vi "Get LV Color.vi"(8 "error in (no error)":errorcluster, 11 "Color in":refnum<class "Color.lvclass">) -> (0 "error out":errorcluster, 2 "Color":u32(colorbox), 3 "Color out":refnum<class "Color.lvclass">)   [LabVIEW 2018, in "Color.lvclass"]
doc: "A method to get the LabVIEW color value corresponding the current color."
uses:
  Color.lvclass
panel:
  # "expressionflow.com"
  # "Copyright (c) 2008 Tomi Maila. All rights reserved."
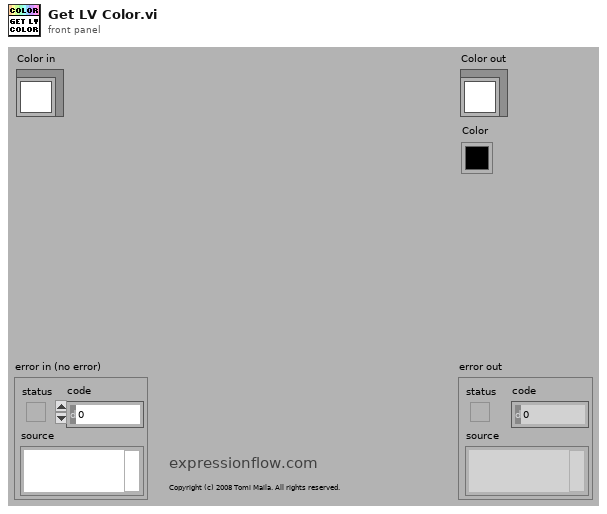
[diagram p1: front panel]
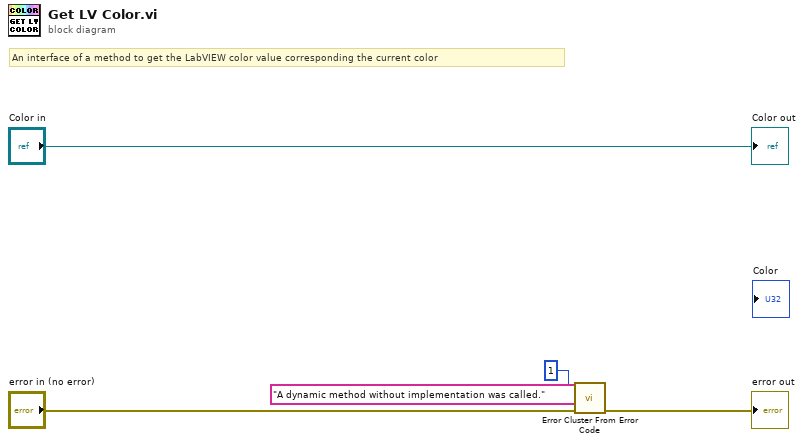
[diagram p0: block diagram]
diagram:
  # "An interface of a method to get the LabVIEW color value corresponding the current color"
  n1 = call <vilib>:"Error Cluster From Error Code.vi"("error in (no error)"="error in (no error)", "error message (\"\")"="A dynamic method without implementation was called." ("error message (\"\")"), "error code (0)"=1) -> ("error out"=→"error out":errorcluster)  [unwired: 6 in]
  "Color out" <- "Color in"
